vi "TUNA forebrain THINK.vi"(5 "MDF in":T1(array[cluster])=[{"Type"=enum."Start", "X"=250, "Y"=250, "Speed"=0, "Behaviors"=enum."Open Water Transit"}, {"Type"=enum."Waypoint", "X"=400, "Y"=100, "Speed"=20, "Behaviors"=enum."P-Wall Follow"}, {"Type"=enum."Waypoint", "X"=250, "Y"=250, "Speed"=20, "Behaviors"=enum."Open Water Transit"}, {"Type"=enum."Waypoint", "X"=250, "Y"=400, "Speed"=20, "Behaviors"=enum."Open Water Transit"}, {"Type"=enum."Waypoint", "X"=100, "Y"=400, "Speed"=20, "Behaviors"=enum."Open Water Transit"}, {"Type"=enum."End", "X"=250, "Y"=250, "Speed"=0, "Behaviors"=enum."Open Water Transit"}], 6 "error in":errorcluster, 7 "Run?":bool=TRUE, 8 "MDF index":i32, 9 "GPS":cluster{"X pos":i32, "Y pos":i32, "Heading":dbl}={"X pos"=250, "Y pos"=250, "Heading"=0.0}) -> (0 "error out":errorcluster, 1 "local Steering\nangle":dbl, 2 "MDF Index out":i32, 3 "Behaviors out":T2, 4 "Complete?":bool=TRUE)   [LabVIEW 2014]
panel:
  out "At Waypoint?":bool
  out "Forebrain Command":T3
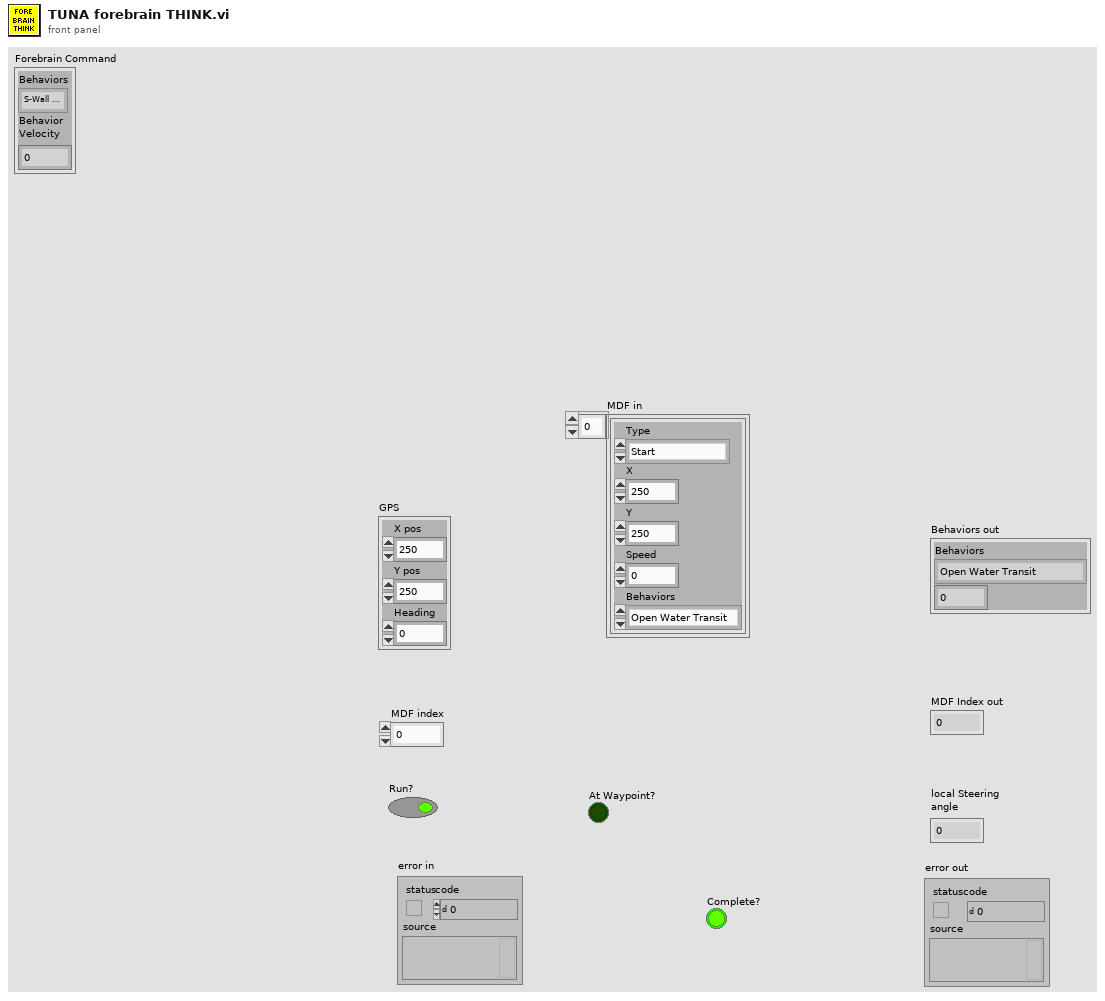
[diagram p1: front panel]
types:
  T1 = cluster{"Type":enum16{"Start", "Waypoint", "End"}, "X":i32, "Y":i32, "Speed":i32, "Behaviors":enum16{"Open Water Transit", "P-Wall Follow", "S-Wall Follow", "Dock"}}[]
  T2 = cluster{"Behaviors":enum16{"Open Water Transit", "P-Wall Follow", "S-Wall Follow", "Dock"}, dbl}
  T3 = cluster{"Behaviors":enum16{"S-Wall Follow", "P-Wall Follow", "Open Water Transit", "Get Unstuck"}, "Behavior\nVelocity":dbl}
  T4 = enum16{"Open Water Transit", "P-Wall Follow", "S-Wall Follow", "Dock"}
  T5 = cluster{"Type":enum16{"Start", "Waypoint", "End"}, "X":i32, "Y":i32, "Speed":i32, "Behaviors":enum16{"Open Water Transit", "P-Wall Follow", "S-Wall Follow", "Dock"}}
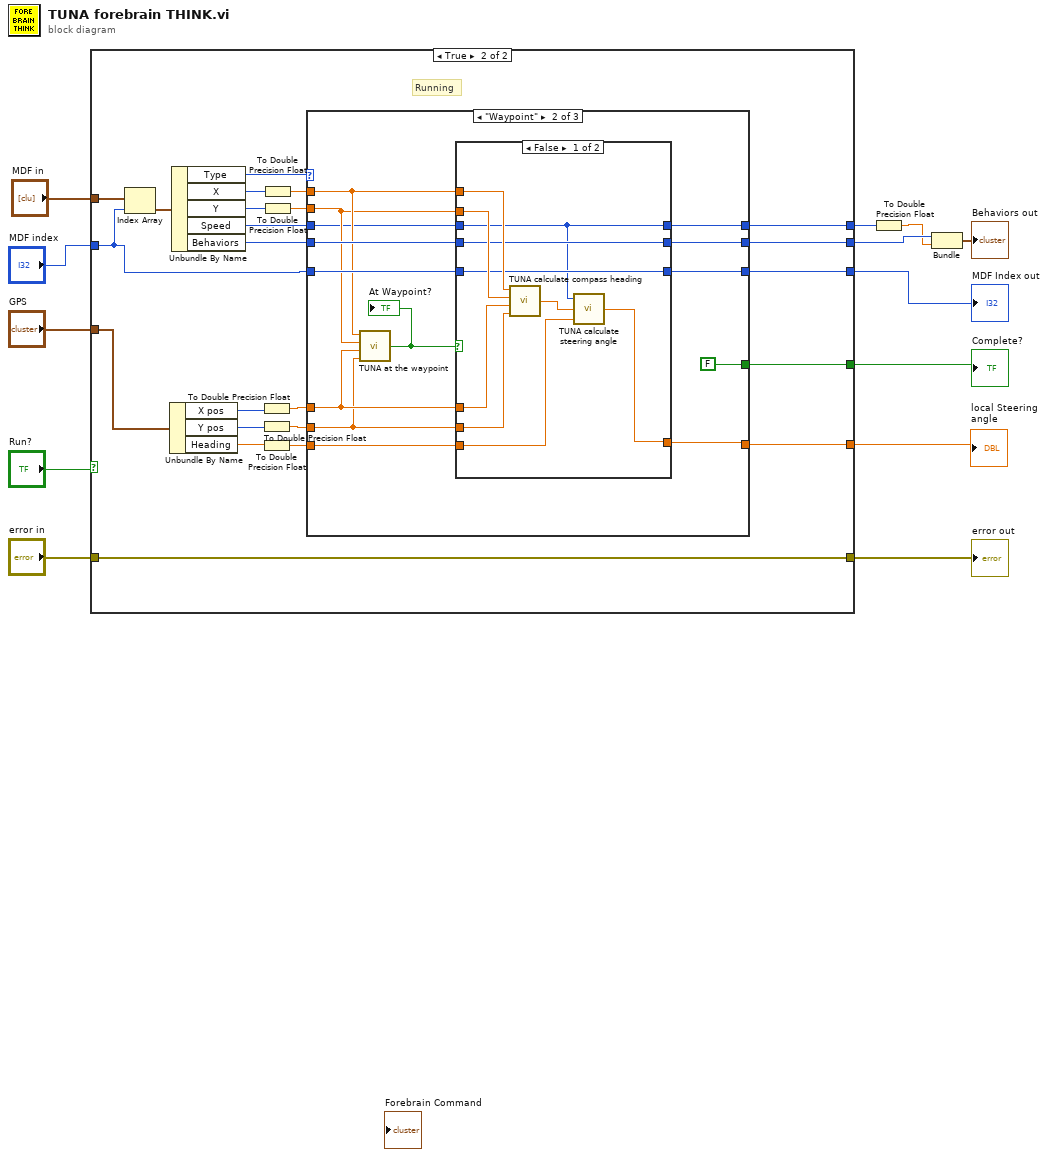
[diagram p0: block diagram]
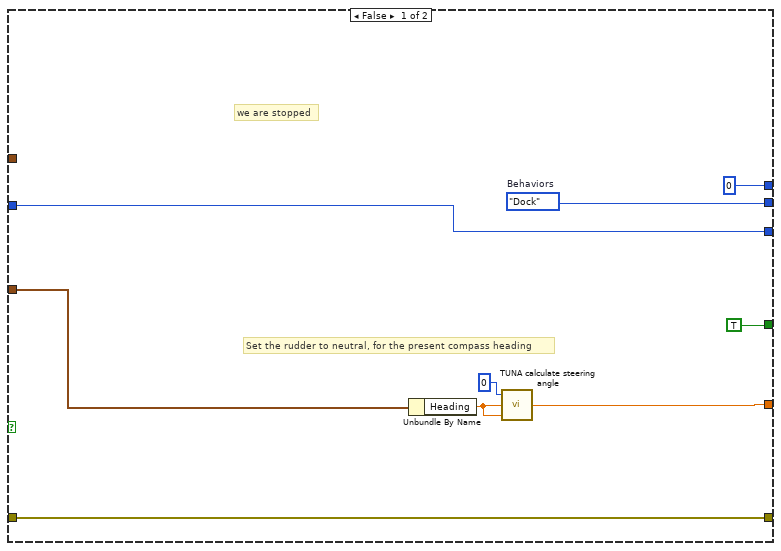
[diagram p2: hidden frame]
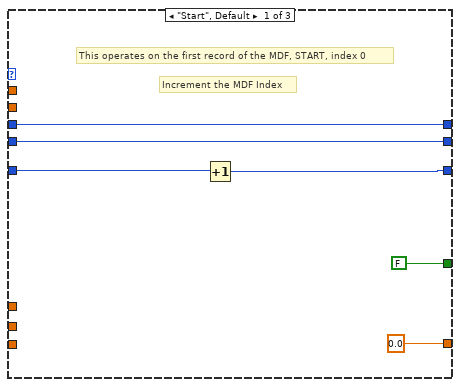
[diagram p3: hidden frame]
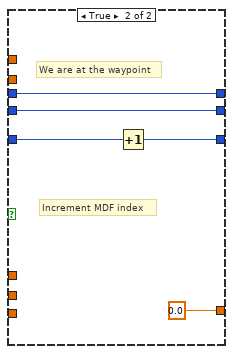
[diagram p4: hidden frame]
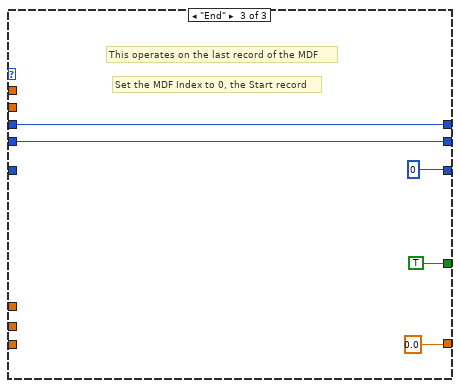
[diagram p5: hidden frame]
diagram:
  n1 = case shown="True" "Run?" {
    tunnel: "MDF in" -> [_ w45]
    tunnel: "MDF index" -> [w18 w30]
    tunnel: "error in" -> [w22 w42]
    tunnel: [w22 w42] -> w11
    tunnel: "GPS" -> [w21 w41]
    tunnel: [w18 w28] -> w8
    tunnel: [w19 w27] -> w7
    tunnel: [0 w25] -> w6
    tunnel: [w16 w24] -> w5
    tunnel: [TRUE w23] -> w2
    frame False {
      w16 = T4."Dock"  # Behaviors
      # "Set the rudder to neutral, for the present compass heading"
      # "we are stopped"
      n2 = Unbundle By Name(w21) -> ("Heading"=w20:dbl)
      n3 = call "TUNA calculate steering angle.vi"("Compass\nheading"=w20, "New heading"=w20, "Speed"=0) -> ("Local Steering Angle"=w19:dbl)
    }
    frame True {
      # "Running"
      n4 = Index Array(array=w45, index=w30) -> (element=w44:T5)
      n5 = Unbundle By Name(w41) -> ("X pos"=w38:i32, "Y pos"=w36:i32, "Heading"=w37:dbl)
      n6 = Unbundle By Name(w44) -> ("Type"=w43:enum16{"Start", "Waypoint", "End"}, "X"=w39:i32, "Y"=w40:i32, "Speed"=w26:i32, "Behaviors"=w29:T4)
      n7 = To Double Precision Float(number=w38) -> (double precision float=w33:dbl)
      n8 = To Double Precision Float(number=w36) -> (double precision float=w32:dbl)
      n9 = To Double Precision Float(number=w37) -> (double precision float=w31:dbl)
      n10 = To Double Precision Float(number=w39) -> (double precision float=w35:dbl)
      n11 = To Double Precision Float(number=w40) -> (double precision float=w34:dbl)
      n12 = case shown="\"Waypoint\"" w43 {
        tunnel: w35 -> [_ w56 _]
        tunnel: w34 -> [_ w55 _]
        tunnel: w33 -> [_ w59 _]
        tunnel: w32 -> [_ w58 _]
        tunnel: w31 -> [_ w57 _]
        tunnel: w30 -> [w49 w62 _]
        tunnel: [w48 w61 0] -> w28
        tunnel: w29 -> [w51 w64 w85]
        tunnel: [w51 w63 w85] -> w24
        tunnel: [0.0 w60 0.0] -> w27
        tunnel: w26 -> [w47 w54 w82]
        tunnel: [w47 w53 w82] -> w25
        tunnel: [FALSE FALSE TRUE] -> w23
        frame "Start", Default {
          # "Increment the MDF Index"
          # "This operates on the first record of the MDF, START, index 0"
          n13 = Increment(x=w49) -> (x+1=w48:i32)
        }
        frame "Waypoint" {
          n14 = call "TUNA at the waypoint.vi"("Y location"=w58, "X location"=w59, "Yof waypoint"=w55, "X of waypoint"=w56) -> ("At Waypoint?"=w65:bool)
          "At Waypoint?" <- w65
          n15 = case shown="False" w65 {
            tunnel: w64 -> [w67 w80]
            tunnel: [w67 w80] -> w63
            tunnel: w62 -> [w68 w79]
            tunnel: [w68 w78] -> w61
            tunnel: [w69 0.0] -> w60
            tunnel: w59 -> [w73 _]
            tunnel: w58 -> [w72 _]
            tunnel: w57 -> [w70 _]
            tunnel: w56 -> [w75 _]
            tunnel: w55 -> [w74 _]
            tunnel: w54 -> [w66 w76]
            tunnel: [w66 w76] -> w53
            frame False {
              n16 = call "TUNA calculate compass heading.vi"("Y Location"=w72, "X Location"=w73, "Waypoint Y"=w74, "Waypoint X"=w75) -> ("Heading"=w71:dbl)
              n17 = call "TUNA calculate steering angle.vi"("Compass\nheading"=w70, "New heading"=w71, "Speed"=w66) -> ("Local Steering Angle"=w69:dbl)
            }
            frame True {
              # "We are at the waypoint"
              # "Increment MDF index"
              n18 = Increment(x=w79) -> (x+1=w78:i32)
            }
          }
        }
        frame "End" {
          # "Set the MDF Index to 0, the Start record"
          # "This operates on the last record of the MDF"
        }
      }
    }
  }
  "error out" <- w11
  "local Steering\nangle" <- w7
  "MDF Index out" <- w8
  "Complete?" <- w2
  n19 = To Double Precision Float(number=w6) -> (double precision float=w4:dbl)
  n20 = Bundle("Behaviors"=w5, w4) -> (→"Behaviors out":T2)  [unwired: 1 in]
